vi "main.vi"() -> ()   [LabVIEW 2013]
uses:
  qwtblvlib/TD Quantity.ctl
  TD GUI Settings.ctl
  qwtblvlib/TD Backend Engine.ctl
  qwtblvlib/TD Algorithm Information.ctl
  qwtblvlib/TD Algorithm Information Input.ctl
  qwtblvlib/TD Algorithm Information Output.ctl
  qwtblvlib/TD Calculation Settings.ctl
  qwtblvlib/TD Uncertainty Calculation Method.ctl
  qwtblvlib/TD Correlation Calculation Settings.ctl
  qwtblvlib/TD DOF Calculation Settings.ctl
  qwtblvlib/TD MCM Calculation Settings.ctl
  qwtblvlib/TD MCM Calculation Method.ctl
  globals.vi
  <vilib>/Utility/xml.llb/Read From XML File(string).vi
  <vilib>/Utility/xml.llb/Write to XML File(string).vi
  qwtblvlib/QWTBLVLib.lvlib
panel:
  in  "show settings":bool
  in  "show algorithms":bool
  in  "show output data":bool
  in  "show input data":bool
  in  "calculate":bool
  in  "about":bool
  out "error out":errorcluster
  in  "quit":bool
  # "simple QWTB GUI"
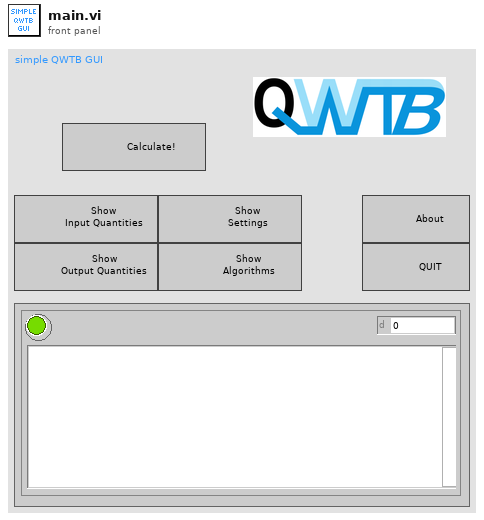
[diagram p1: front panel]
types:
  T1 = typedef "QWTBLVLib.lvlib/TD Quantity.ctl" = cluster{"Name":string, "Value":dbl[][], "Uncertainty":dbl[][], "Degrees of Freedom":dbl[][], "Correlation":dbl[][], "Randomized uncertainty":dbl[][]}
  T2 = typedef "QWTBLVLib.lvlib/TD Calculation Settings.ctl" = cluster{"Strict":bool, "Verbose":bool, "Uncertainty Calculation Method":T3, "Correlations":T4, "Degrees of Freedom":T5, "MCM Calculation Settings":T6}
  T3 = typedef "QWTBLVLib.lvlib/TD Uncertainty Calculation Method.ctl" = enum16{"none", "GUF", "MCM"}
  T4 = typedef "QWTBLVLib.lvlib/TD Correlation Calculation Settings.ctl" = cluster{"Required":bool, "Generate":bool}
  T5 = typedef "QWTBLVLib.lvlib/TD DOF Calculation Settings.ctl" = cluster{"Required":bool, "Generate":bool}
  T6 = typedef "QWTBLVLib.lvlib/TD MCM Calculation Settings.ctl" = cluster{"Repeats":i32, "Verbose":bool, "Parallelization method":T7, "Processors":i32, "Temporary directory":string, "Randomize":bool}
  T7 = typedef "QWTBLVLib.lvlib/TD MCM Calculation Method.ctl" = enum16{"Single Core", "Multi Core", "Multi Station"}
  T8 = typedef "QWTBLVLib.lvlib/TD Algorithm Information.ctl" = cluster{"ID":string, "Name":string, "Description":string, "Citation":string, "Remarks":string, "License":string, "Inputs":T9[], "Outputs":T10[], "Provides GUF":bool, "Provides MCM":bool, "Full path":string}
  T9 = typedef "QWTBLVLib.lvlib/TD Algorithm Information Input.ctl" = cluster{"Name":string, "Description":string, "Alternative":i32, "Optional":i32, "Parameter":i32}
  T10 = typedef "QWTBLVLib.lvlib/TD Algorithm Information Output.ctl" = cluster{"Name":string, "Description":string}
  T11 = typedef "TD GUI Settings.ctl" = cluster{"Backend engine":T12, "QWTB Folder Path":path}
  T12 = typedef "QWTBLVLib.lvlib/TD Backend Engine.ctl" = enum16{"Matlab by Script node", "GNU Octave by GOLPI"}
  T13 = enum32{"Invalid", "Standard", "Closed", "Hidden", "Minimized", "Maximized"}
  T14 = cluster{"Calculation Settings":T2, "GUI Settings":T11, "Data In":T1[], "Available Algorithms":T8[], "Current Algorithm":T8, "Data Out":T1[]}
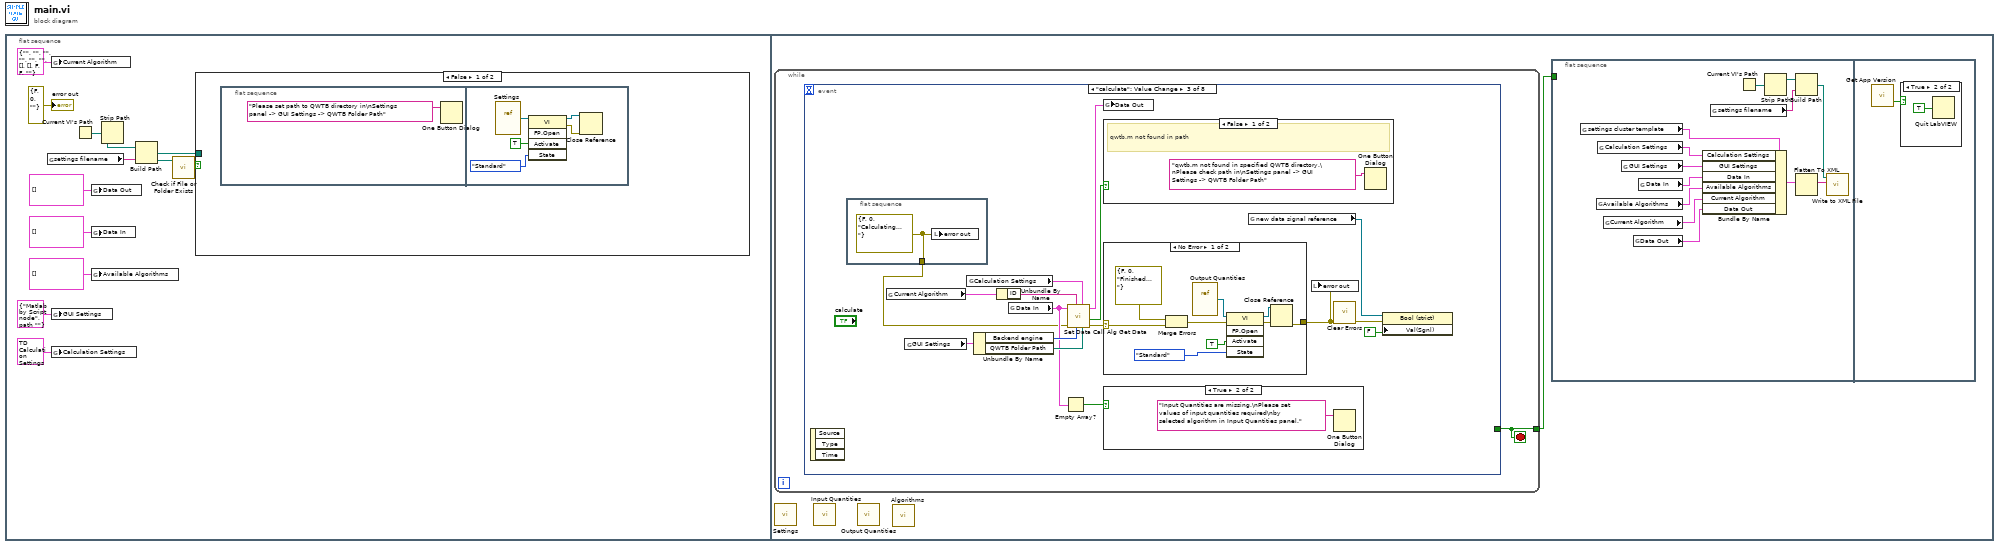
[diagram p0: block diagram]
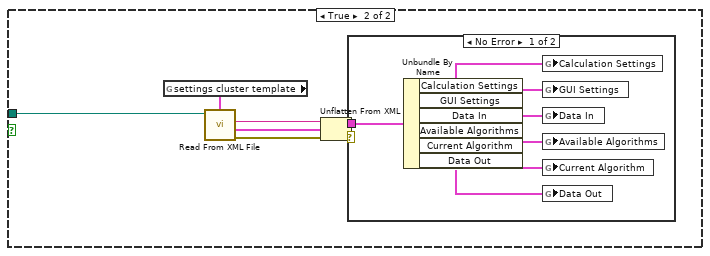
[diagram p2: hidden frame]
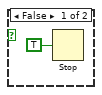
[diagram p4: hidden frame]
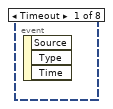
[diagram p5: hidden frame]
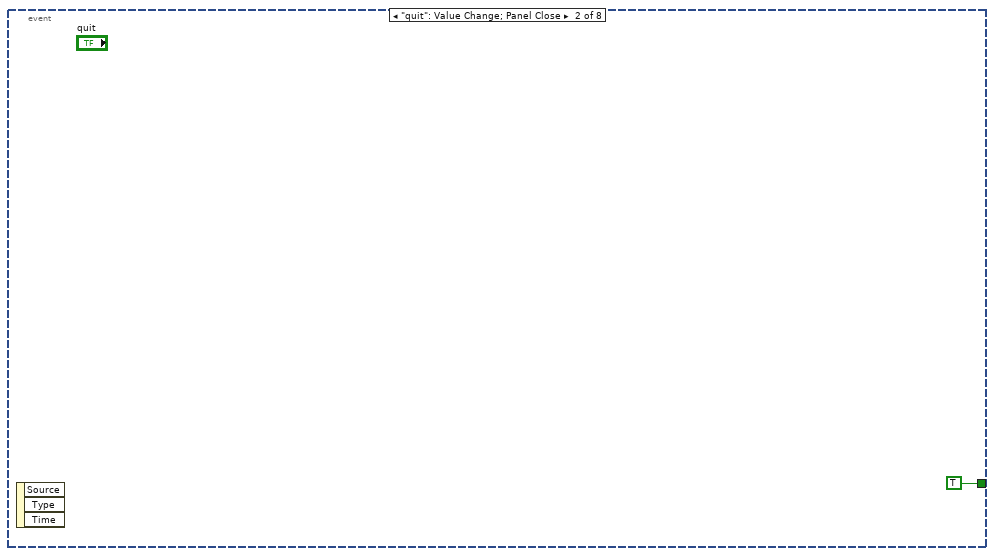
[diagram p6: hidden frame]
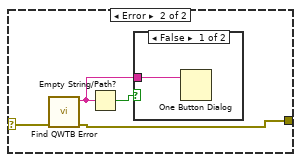
[diagram p9: hidden frame]
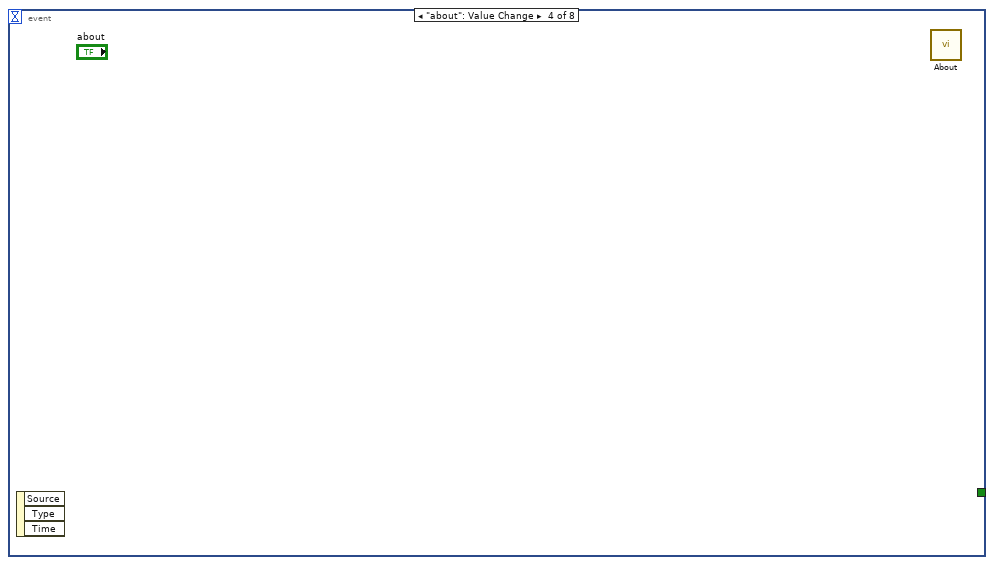
[diagram p11: hidden frame]
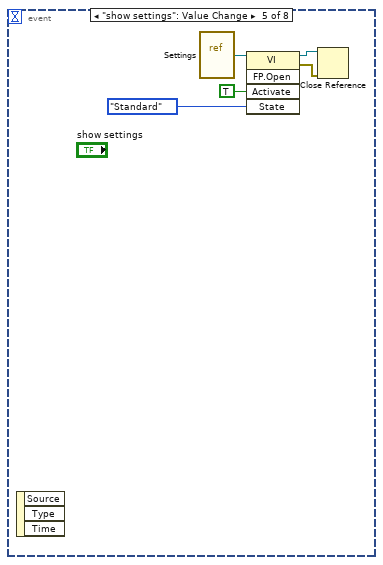
[diagram p12: hidden frame]
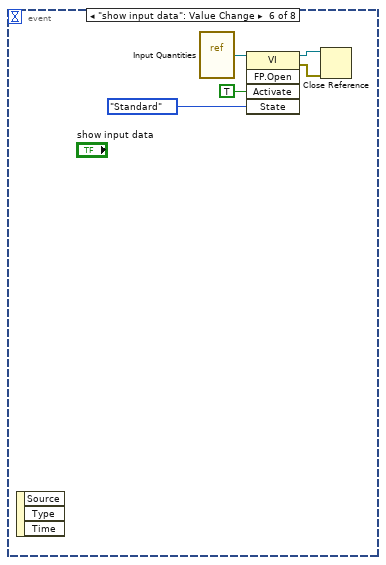
[diagram p13: hidden frame]
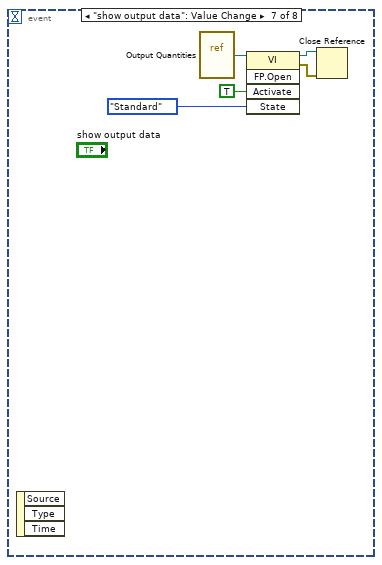
[diagram p14: hidden frame]
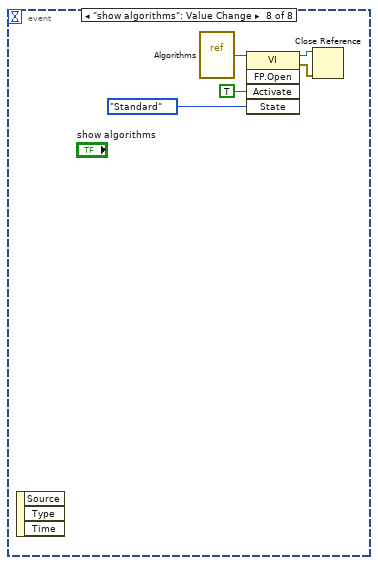
[diagram p15: hidden frame]
diagram:
  n1 = flat-sequence {
    frame #0 {
      n2 = global read "globals.vi" "settings filename"() -> (w7:string)
      n3 = global write "globals.vi" "Current Algorithm"(T8 {"ID"="", "Name"="", "Description"="", "Citation"="", "Remarks"="", "License"="", "Inputs"=[], "Outputs"=[], "Provides GUF"=FALSE, "Provides MCM"=FALSE, "Full path"=""} ("Current Algorithm")) -> ()
      n4 = global write "globals.vi" "GUI Settings"(T11 {"Backend engine"=enum."Matlab by Script node", "QWTB Folder Path"=path ""} ("GUI Settings")) -> ()
      n5 = global write "globals.vi" "Calculation Settings"(T2 {"Strict"=FALSE, "Verbose"=TRUE, "Uncertainty Calculation Method"=enum."none", "Correlations"={"Required"=FALSE, "Generate"=FALSE}, "Degrees of Freedom"={"Required"=FALSE, "Generate"=FALSE}, "MCM Calculation Settings"={"Repeats"=100, "Verbose"=TRUE, "Parallelization method"=enum."Single Core", "Processors"=0, "Temporary directory"=".", "Randomize"=TRUE}} ("Calculation Settings")) -> ()
      n6 = Current VI's Path() -> (path=w4:path)
      n7 = global write "globals.vi" "Data Out"(T1[] [] ("Data Out")) -> ()
      n8 = global write "globals.vi" "Data In"(T1[] []) -> ()
      n9 = global write "globals.vi" "Available Algorithms"(T8[] [] ("Available Algorithms")) -> ()
      n10 = Strip Path(path=w4) -> (stripped path=w3:path)  [unwired: 1 out]
      n11 = Build Path(base path=w3, name or relative path=w7) -> (appended path=w5:path)
      n12 = call <vilib>:"Check if File or Folder Exists.vi"("path"=w5) -> ("file or folder exists?"=w6:bool)  [unwired: 8 in, 2 out]
      n13 = case shown="False" w6 {
        tunnel: w5 -> [_ w20]
        frame False {
          n14 = flat-sequence {
            frame #0 {
              n15 = One Button Dialog(message="Please set path to QWTB directory in\nSettings panel -> GUI Settings -> QWTB Folder Path") -> ()  [unwired: 1 in, 1 out]
            }
            frame #1 {
              n16 = vi-ref "Settings.vi"() -> (w16:refnum<vi>)
              n17 = invoke class="VI" method="FP.Open"(reference=w16, "Activate"=TRUE ("Activate?"), "State"=T13."Standard") -> (reference out=w14:refnum<vi>, error out=w15:errorcluster)  [unwired: 2 in, 3 out]
              n18 = Close Reference(reference=w14, error in (no error)=w15) -> ()  [unwired: 1 out]
            }
          }
        }
        frame True {
          n19 = global read "globals.vi" "settings cluster template"() -> (w19:T14)
          n20 = call-poly <vilib>:"Read From XML File.vi"("XML File Path"=w20) -> ("error out"=w23:errorcluster, "XML Elements"=w24:string)  [unwired: 8 in, 1 out]
          n21 = Unflatten From XML(xml string=w24, type=w19, error in (no error)=w23) -> (value=w21:T14, error out=w22:errorcluster)
          n22 = case shown="No Error" w22 {
            tunnel: w21 -> [w31 _]
            frame No Error {
              n23 = Unbundle By Name(w31) -> ("Calculation Settings"=w30:T2, "GUI Settings"=w29:T11, "Data In"=w28:T1[], "Available Algorithms"=w27:T8[], "Current Algorithm"=w26:T8, "Data Out"=w25:T1[])
              n24 = global write "globals.vi" "Calculation Settings"(w30) -> ()
              n25 = global write "globals.vi" "GUI Settings"(w29) -> ()
              n26 = global write "globals.vi" "Data In"(w28) -> ()
              n27 = global write "globals.vi" "Available Algorithms"(w27) -> ()
              n28 = global write "globals.vi" "Current Algorithm"(w26) -> ()
              n29 = global write "globals.vi" "Data Out"(w25) -> ()
            }
            frame Error {
            }
          }
        }
      }
      "error out" <- errorcluster {"status"=FALSE, "code"=0, "source"=""} ("error constant")
    }
    frame #1 {
      n30 = while {
        tunnel: [w49] -> w32
        stop <- w49 stop-if-true
        n31 = event shown="[2] \"calculate\": Value Change" {
          selector: _ -> [_ _ _ _ _ _ _ _]
          dyn-events: _ -> [_ _ _ _ _ _ _ _]
          timeout: _ -> [_ _ _ _ _ _ _ _]
          tunnel: [_ TRUE _ _ _ _ _ _] -> w49
          event Timeout {
            n32 = event-data() -> ()  [unwired: 1 in, 3 out]
          }
          event "quit": Value Change; Panel Close {
            n33 = event-data() -> ()  [unwired: 1 in, 3 out]
          }
          event "calculate": Value Change {
            n34 = event-data() -> ()  [unwired: 1 in, 3 out]
            n35 = flat-sequence {
              tunnel: [w67] -> w51
              frame #0 {
                w67 = errorcluster {"status"=FALSE, "code"=0, "source"="Calculating..."} ("error out")
                n36 = local write "error out"(w67) -> ()
              }
            }
            n37 = global read "globals.vi" "Current Algorithm"() -> (w58:T8)
            n38 = global read "globals.vi" "GUI Settings"() -> (w62:T11)
            n39 = global read "globals.vi" "Calculation Settings"() -> (w63:T2)
            n40 = Unbundle By Name(w62) -> ("Backend engine"=w61:T12, "QWTB Folder Path"=w60:path)
            n41 = Unbundle By Name(w58) -> ("ID"=w57:string)
            n42 = global read "globals.vi" "Data In"() -> (w53:T1[])
            n43 = Empty Array?(array=w53) -> (empty?=w52:bool)
            n44 = call "Set Data Call Alg Get Data.vi"("QWTB Folder Path"=w60, "Calculation Settings"=w63, "Backend engine"=w61, "Algorithm ID"=w57, "error in"=w51, "Data In"=w53) -> ("error out"=w56:errorcluster, "qwtb.m found in path"=w54:bool, "Data Out"=w66:T1[])  [unwired: 3 in]
            n45 = global write "globals.vi" "Data Out"(w66) -> ()
            n46 = case shown="False" w54 {
              frame False {
                # "qwtb.m not found in path"
                n47 = One Button Dialog(message="qwtb.m not found in specified QWTB directory.\nPlease check path in\nSettings panel -> GUI Settings -> QWTB Folder Path") -> ()  [unwired: 1 in, 1 out]
              }
              frame True {
              }
            }
            n48 = case shown="No Error" w56 {
              selector: w56 -> [w75 w82]
              tunnel: [w71 w81] -> w55
              frame No Error {
                n49 = Merge Errors(errorcluster {"status"=FALSE, "code"=0, "source"="Finished..."} ("error out"), w75) -> (w73:errorcluster)
                n50 = vi-ref "Output Quantities.vi"() -> (w78:refnum<vi>)
                n51 = invoke class="VI" method="FP.Open"(reference=w78, error in=w73, "Activate"=TRUE ("Activate?"), "State"=T13."Standard") -> (reference out=w70:refnum<vi>, error out=w72:errorcluster)  [unwired: 1 in, 3 out]
                n52 = Close Reference(reference=w70, error in (no error)=w72) -> (error out=w71:errorcluster)
              }
              frame Error {
                n53 = call "Find QWTB Error.vi"("error in (no error)"=w82) -> ("error out"=w81:errorcluster, "QWTB error\n(empty string)"=w79:string)  [unwired: 8 in, 1 out]
                n54 = Empty String/Path?(string/path=w79) -> (empty?=w80:bool)
                n55 = case shown="False" w80 {
                  tunnel: w79 -> [w83 _]
                  frame False {
                    n56 = One Button Dialog(message=w83) -> ()  [unwired: 1 in, 1 out]
                  }
                  frame True {
                  }
                }
              }
            }
            n57 = case shown="True" w52 {
              frame False {
              }
              frame True {
                n58 = One Button Dialog(message="Input Quantities are missing.\nPlease set values of input quantities required\nby selected algorithm in Input Quantities panel.") -> ()  [unwired: 1 in, 1 out]
              }
            }
            n59 = global read "globals.vi" "new data signal reference"() -> (w65:refnum<vi>)
            n60 = local write "error out"(w55) -> ()
            n61 = call <vilib>:"Clear Errors.vi"("error in (no error)"=w55) -> ("error out"=w59:errorcluster)  [unwired: 6 in]
            n62 = property class="Bool (strict)"(reference=w65, error in=w59, "Val(Sgnl)"=FALSE ("Value (Signaling)")) -> ()  [unwired: 2 out]
          }
          event "about": Value Change {
            n63 = event-data() -> ()  [unwired: 1 in, 3 out]
            n64 = call "About.vi"() -> ()  [unwired: 1 in]
          }
          event "show settings": Value Change {
            n65 = event-data() -> ()  [unwired: 1 in, 3 out]
            n66 = vi-ref "Settings.vi"() -> (w88:refnum<vi>)
            n67 = invoke class="VI" method="FP.Open"(reference=w88, "Activate"=TRUE ("Activate?"), "State"=T13."Standard") -> (reference out=w84:refnum<vi>, error out=w85:errorcluster)  [unwired: 2 in, 3 out]
            n68 = Close Reference(reference=w84, error in (no error)=w85) -> ()  [unwired: 1 out]
          }
          event "show input data": Value Change {
            n69 = event-data() -> ()  [unwired: 1 in, 3 out]
            n70 = vi-ref "Input Quantities.vi"() -> (w93:refnum<vi>)
            n71 = invoke class="VI" method="FP.Open"(reference=w93, "Activate"=TRUE ("Activate?"), "State"=T13."Standard") -> (reference out=w89:refnum<vi>, error out=w90:errorcluster)  [unwired: 2 in, 3 out]
            n72 = Close Reference(reference=w89, error in (no error)=w90) -> ()  [unwired: 1 out]
          }
          event "show output data": Value Change {
            n73 = event-data() -> ()  [unwired: 1 in, 3 out]
            n74 = vi-ref "Output Quantities.vi"() -> (w98:refnum<vi>)
            n75 = invoke class="VI" method="FP.Open"(reference=w98, "Activate"=TRUE ("Activate?"), "State"=T13."Standard") -> (reference out=w94:refnum<vi>, error out=w95:errorcluster)  [unwired: 2 in, 3 out]
            n76 = Close Reference(reference=w94, error in (no error)=w95) -> ()  [unwired: 1 out]
          }
          event "show algorithms": Value Change {
            n77 = event-data() -> ()  [unwired: 1 in, 3 out]
            n78 = vi-ref "Algorithms.vi"() -> (w103:refnum<vi>)
            n79 = invoke class="VI" method="FP.Open"(reference=w103, "Activate"=TRUE ("Activate?"), "State"=T13."Standard") -> (reference out=w100:refnum<vi>, error out=w99:errorcluster)  [unwired: 2 in, 3 out]
            n80 = Close Reference(reference=w100, error in (no error)=w99) -> ()  [unwired: 1 out]
          }
        }
      }
      n81 = call "Settings.vi"() -> ()  [unwired: 12 in]
      n82 = call "Input Quantities.vi"() -> ()  [unwired: 12 in]
      n83 = call "Output Quantities.vi"() -> ()  [unwired: 12 in]
      n84 = call "Algorithms.vi"() -> ()  [unwired: 12 in]
      n85 = flat-sequence {
        tunnel: w32 -> [_]
        frame #0 {
          n86 = global read "globals.vi" "settings cluster template"() -> (w38:T14)
          n87 = global read "globals.vi" "Available Algorithms"() -> (w42:T8[])
          n88 = global read "globals.vi" "Calculation Settings"() -> (w45:T2)
          n89 = global read "globals.vi" "Current Algorithm"() -> (w41:T8)
          n90 = global read "globals.vi" "GUI Settings"() -> (w44:T11)
          n91 = global read "globals.vi" "Data Out"() -> (w40:T1[])
          n92 = global read "globals.vi" "Data In"() -> (w43:T1[])
          n93 = Bundle By Name(cluster=w38, "Calculation Settings"=w45, "GUI Settings"=w44, "Data In"=w43, "Available Algorithms"=w42, "Current Algorithm"=w41, "Data Out"=w40) -> (w39:T14)
          n94 = global read "globals.vi" "settings filename"() -> (w36:string)
          n95 = Current VI's Path() -> (path=w34:path)
          n96 = Strip Path(path=w34) -> (stripped path=w33:path)  [unwired: 1 out]
          n97 = Build Path(base path=w33, name or relative path=w36) -> (appended path=w37:path)
          n98 = Flatten To XML(anything=w39) -> (xml string=w35:string)
          n99 = call-poly <vilib>:"Write to XML File.vi"("XML Input"=w35, "XML File Path"=w37) -> ()  [unwired: 7 in, 3 out]
        }
        frame #1 {
          n100 = call "Get App Version.vi"() -> ("runtime"=w46:bool)  [unwired: 1 out]
          n101 = case shown="True" w46 {
            frame False {
              n102 = Stop(stop? (T)=TRUE) -> ()
            }
            frame True {
              n103 = Quit LabVIEW(quit? (T)=TRUE) -> ()
            }
          }
        }
      }
    }
  }
